vi "NIFPGA-MCS.contents.vi"   [LabVIEW 2014, in "NIFPGA-MCS.lvlib"]
doc: "Loads all VIs into memory required for building an application"
uses:
  NIFPGA-MCS.lvlib
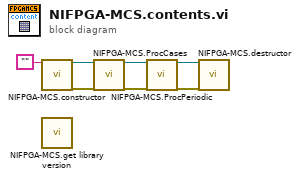
[diagram p0: block diagram]
diagram:
  n1 = call "NIFPGA-MCS.constructor.vi"("name"="") -> ("i ref out"=w7:refnum<vi>, "error out"=w3:errorcluster)  [unwired: 16 in, 1 out]
  n2 = call "NIFPGA-MCS.get library version.vi"() -> ()  [unwired: 1 in, 1 out]
  n3 = call "NIFPGA-MCS.ProcCases.vi"("i ref in"=w7, "error in (no error)"=w3) -> ("i ref out"=w6:refnum<vi>, "error out"=w2:errorcluster)  [unwired: 15 in, 1 out]
  n4 = call "NIFPGA-MCS.ProcPeriodic.vi"("i ref in"=w6, "error in (no error)"=w2) -> ("i ref out"=w5:refnum<vi>, "error out"=w1:errorcluster)  [unwired: 15 in, 1 out]
  n5 = call "NIFPGA-MCS.destructor.vi"("i ref in"=w5, "error in (no error)"=w1) -> ()  [unwired: 17 in, 1 out]
